vi "USB6343_Control_v1.6.2.vi"(8 "error in":errorcluster caption="错误输出", 10 "interface":T2, 11 "tasks":T3) -> ()   [LabVIEW 2013]
uses:
  <vilib>/DAQmx/read.llb/DAQmx Read (Analog 1D DBL NChan 1Samp).vi
  <vilib>/DAQmx/read.llb/DAQmx Read (Digital 1D Bool NChan 1Samp 1Line).vi
  <vilib>/DAQmx/read.llb/DAQmx Read (Counter DBL 1Chan 1Samp).vi
  <vilib>/DAQmx/write.llb/DAQmx Write (Digital 1D Bool NChan 1Samp 1Line).vi
  <vilib>/DAQmx/write.llb/DAQmx Write (Analog 1D DBL NChan 1Samp).vi
  <vilib>/DAQmx/miscellaneous.llb/DAQmx Fill In Error Info.vi
  <vilib>/DAQmx/configure/timing.llb/DAQmx Timing (Implicit).vi
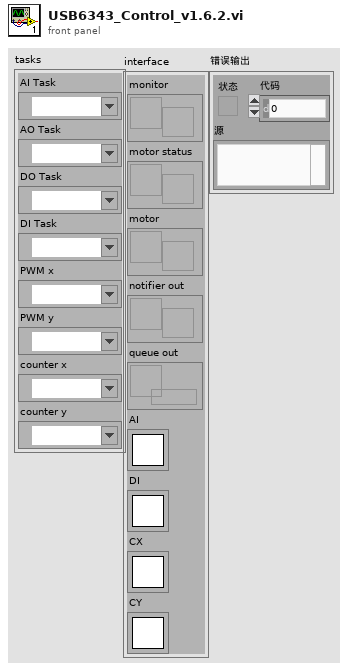
[diagram p1: front panel]
types:
  T1 = typedef "Semaphore RefNum" = refnum<k1>
  T2 = cluster{"monitor":refnum<user-event>, "motor status":refnum<user-event>, "motor":refnum<user-event>, "notifier out":refnum<notifier>, "queue out":refnum<queue>, "AI":T1, "DI":T1, "CX":T1, "CY":T1}
  T3 = cluster{"AI Task":refnum<k21>, "AO Task":refnum<k21>, "DO Task":refnum<k21>, "DI Task":refnum<k21>, "PWM x":refnum<k21>, "PWM y":refnum<k21>, "counter x":refnum<k21>, "counter y":refnum<k21>}
  T4 = cluster{"cmd":string, "channel":i32, "value":dbl, "on/off":bool, "return value":refnum<vi>}
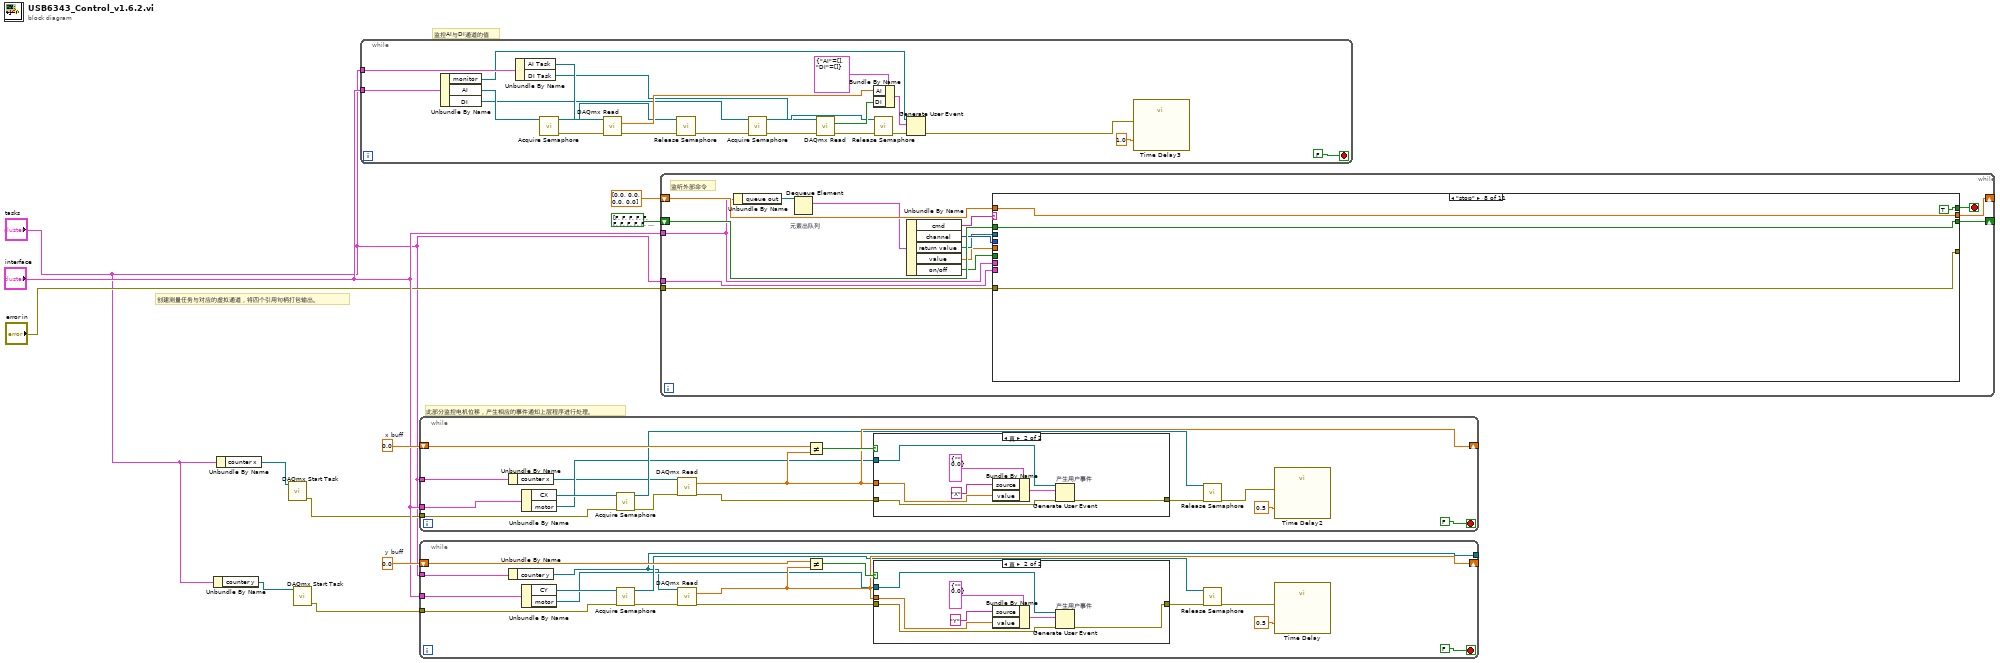
[diagram p0: block diagram]
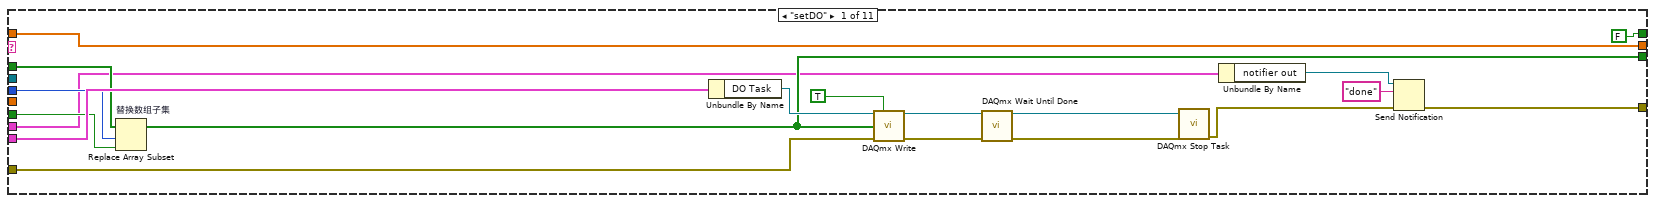
[diagram p4: hidden frame]
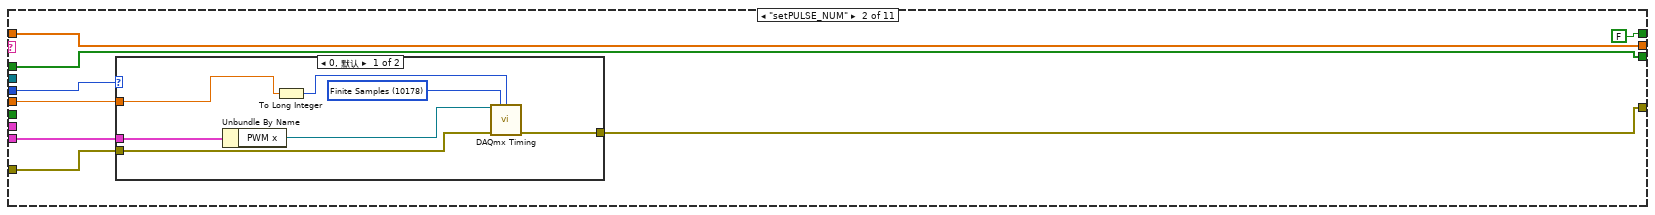
[diagram p5: hidden frame]
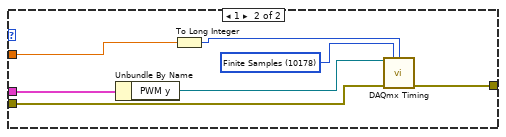
[diagram p6: hidden frame]
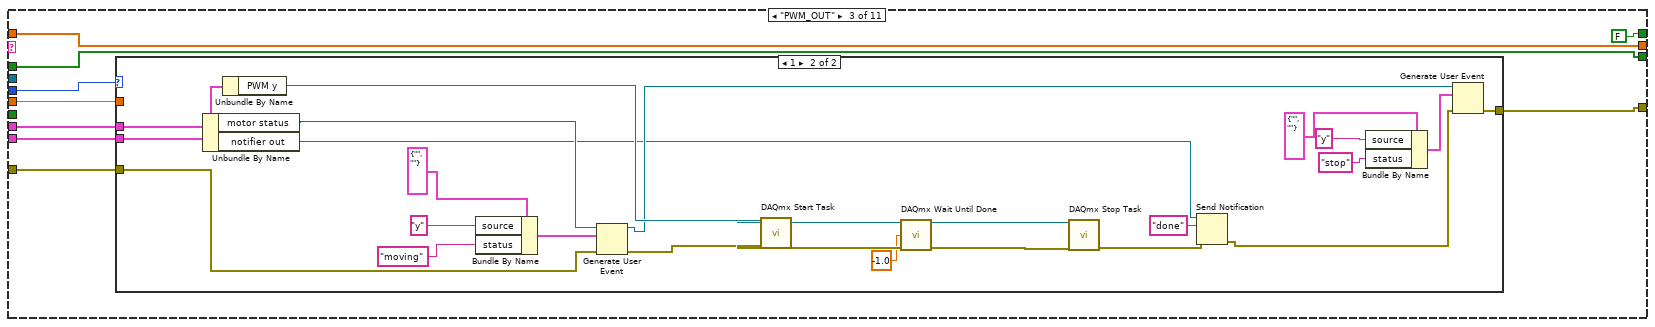
[diagram p7: hidden frame]
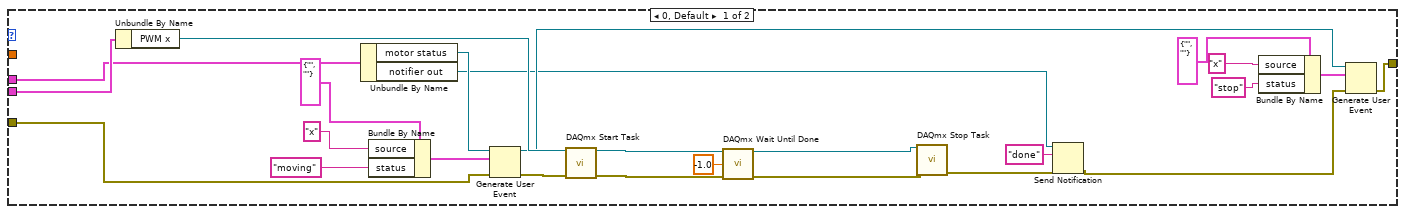
[diagram p8: hidden frame]
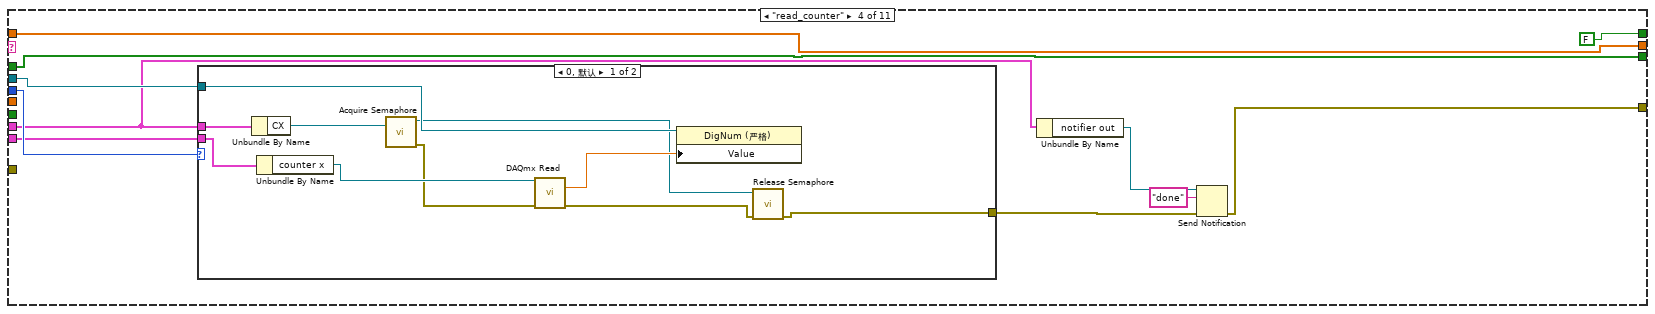
[diagram p9: hidden frame]
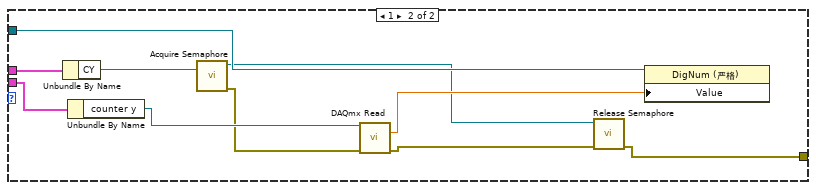
[diagram p10: hidden frame]
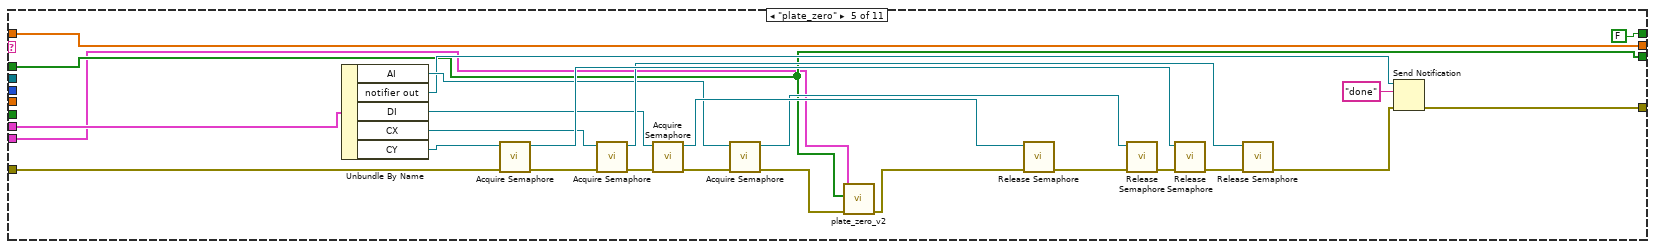
[diagram p11: hidden frame]
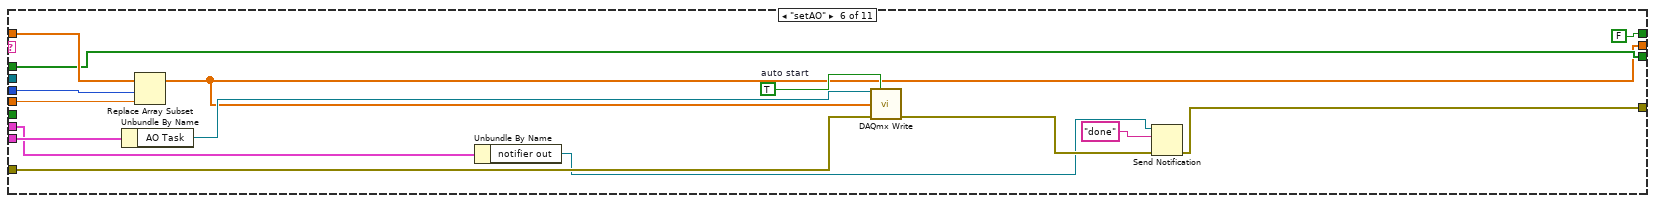
[diagram p12: hidden frame]
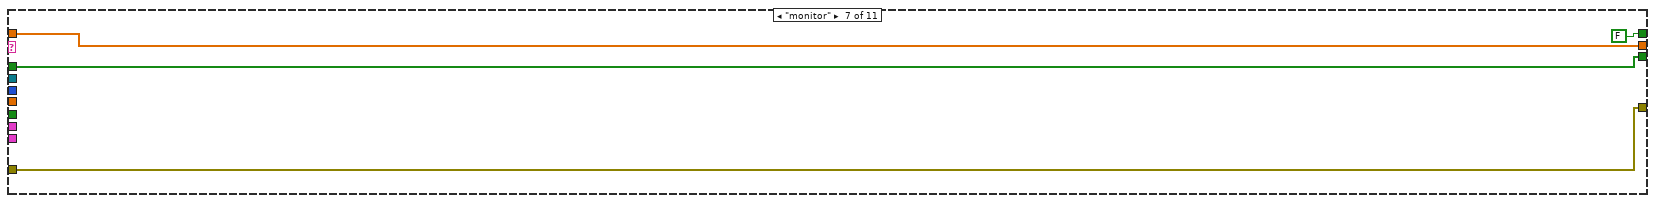
[diagram p13: hidden frame]
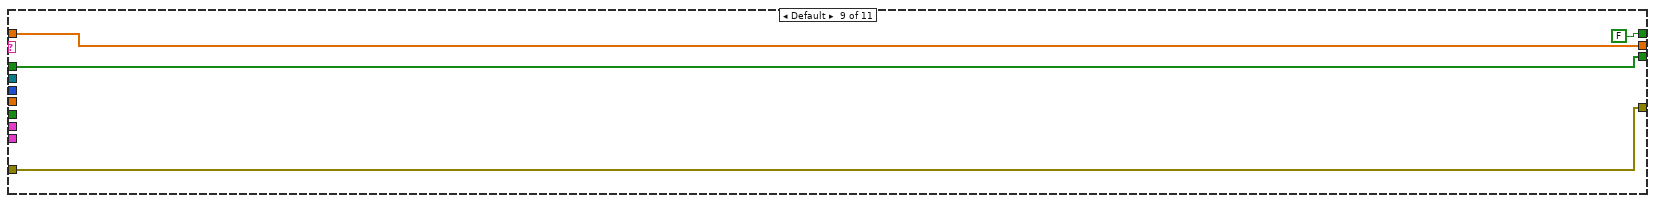
[diagram p14: hidden frame]
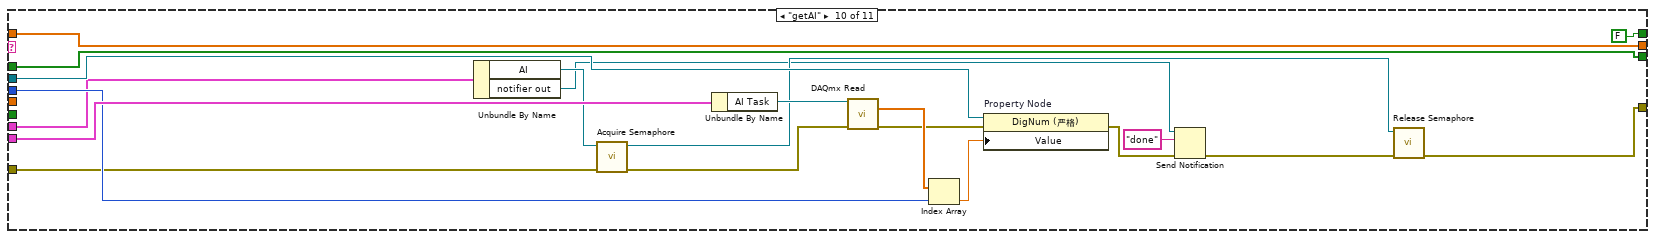
[diagram p15: hidden frame]
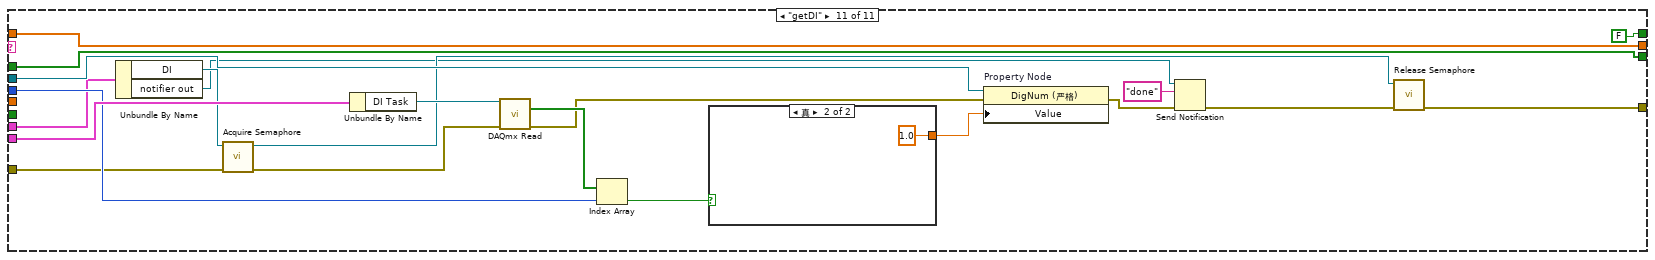
[diagram p16: hidden frame]
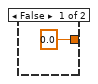
[diagram p17: hidden frame]
diagram:
  w8 = 0.0  # x buff
  w9 = 0.0  # y buff
  # "监控AI与DI通道的值"
  # "此部分监控电机位移，产生相应的事件通知上层程序进行处理。"
  # "创建测量任务与对应的虚拟通道，将四个引用句柄打包输出。"
  n1 = Unbundle By Name("tasks") -> ("counter y"=w1:refnum<k21>)
  n2 = Unbundle By Name("tasks") -> ("counter x"=w3:refnum<k21>)
  n3 = call <vilib>:"DAQmx Start Task.vi"("task/channels in"=w3) -> ("error out"=w4:errorcluster)  [unwired: 13 in, 1 out]
  n4 = call <vilib>:"DAQmx Start Task.vi"("task/channels in"=w1) -> ("error out"=w5:errorcluster)  [unwired: 13 in, 1 out]
  n5 = while {
    tunnel: "tasks" -> [w31]
    tunnel: "interface" -> [w16]
    stop <- FALSE stop-if-true
    n6 = Unbundle By Name(w16) -> ("monitor"=w15:refnum<user-event>, "AI"=w14:T1, "DI"=w13:T1)
    n7 = Unbundle By Name(w31) -> ("AI Task"=w32:refnum<k21>, "DI Task"=w12:refnum<k21>)
    n8 = call <vilib>:"Acquire Semaphore.vi"("semaphore"=w14) -> ("error out"=w17:errorcluster, "semaphore out"=w19:T1)  [unwired: 4 in, 1 out]
    n9 = call-poly <vilib>:"DAQmx Read.vi"("task/channels in"=w32, "error in"=w17) -> ("data"=w29:dbl[], "error out"=w24:errorcluster)  [unwired: 11 in, 1 out]
    n10 = call <vilib>:"Release Semaphore.vi"("error in (no error)"=w24, "semaphore"=w19) -> ("error out"=w23:errorcluster)  [unwired: 4 in, 1 out]
    n11 = call <vilib>:"Acquire Semaphore.vi"("error in (no error)"=w23, "semaphore"=w13) -> ("error out"=w22:errorcluster, "semaphore out"=w18:T1)  [unwired: 3 in, 1 out]
    n12 = call-poly <vilib>:"DAQmx Read.vi"("task/channels in"=w12, "error in"=w22) -> ("data"=w28:bool[], "error out"=w21:errorcluster)  [unwired: 11 in, 1 out]
    n13 = Bundle By Name(cluster=cluster{"AI":dbl[], "DI":bool[]} {"AI"=[], "DI"=[]} ("event data"), "AI"=w29, "DI"=w28) -> (w25:cluster{"AI":dbl[], "DI":bool[]})
    n14 = call <vilib>:"Release Semaphore.vi"("error in (no error)"=w21, "semaphore"=w18) -> ("error out"=w20:errorcluster)  [unwired: 4 in, 1 out]
    n15 = Generate User Event(user event=w15, event data cluster=w25, error in=w20) -> (error out=w27:errorcluster)  [unwired: 1 in, 1 out]
    n16 = call "Time Delay3"("error in (no error)"=w27, "Delay Time (s)"=1.0) -> ()  [unwired: 9 in, 1 out]
  }
  n17 = while {
    shift-right: [w45] -> _
    shift-left: w8 -> [w49]
    tunnel: "interface" -> [w39]
    tunnel: "tasks" -> [w36]
    tunnel: w4 -> [w34]
    stop <- FALSE stop-if-true
    n18 = Unbundle By Name(w36) -> ("counter x"=w35:refnum<k21>)
    n19 = Unbundle By Name(w39) -> ("CX"=w38:T1, "motor"=w37:refnum<user-event>)
    n20 = call <vilib>:"Acquire Semaphore.vi"("error in (no error)"=w34, "semaphore"=w38) -> ("error out"=w44:errorcluster, "semaphore out"=w41:T1)  [unwired: 3 in, 1 out]
    n21 = call-poly <vilib>:"DAQmx Read.vi"("task/channels in"=w35, "error in"=w44) -> ("data"=w45:dbl, "error out"=w47:errorcluster)  [unwired: 11 in, 1 out]
    n22 = Not Equal?(x=w49, y=w45) -> (x != y?=w48:bool)
    n23 = case shown="真" w48 {
      tunnel: w45 -> [_ w51]
      tunnel: w47 -> [w50 w54]
      tunnel: [w50 w53] -> w43
      tunnel: w37 -> [_ w52]
      frame False {
      }
      frame True {
        n24 = Bundle By Name(cluster=cluster{"source":string, "value":dbl} {"source"="", "value"=0.0} ("事件数据"), "source"="X", "value"=w51) -> (w55:cluster{"source":string, "value":dbl})
        n25 = Generate User Event "产生用户事件"(user event=w52, event data cluster=w55, error in=w54) -> (error out=w53:errorcluster)  [unwired: 1 in, 1 out]
      }
    }
    n26 = call <vilib>:"Release Semaphore.vi"("error in (no error)"=w43, "semaphore"=w41) -> ("error out"=w42:errorcluster)  [unwired: 4 in, 1 out]
    n27 = call "Time Delay2"("error in (no error)"=w42, "Delay Time (s)"=0.5) -> ()  [unwired: 9 in, 1 out]
  }
  n28 = while {
    tunnel: [w59] -> _
    shift-right: [w69] -> _
    shift-left: w9 -> [w73]
    tunnel: "interface" -> [w63]
    tunnel: "tasks" -> [w60]
    tunnel: w5 -> [w58]
    stop <- FALSE stop-if-true
    n29 = Unbundle By Name(w60) -> ("counter y"=w59:refnum<k21>)
    n30 = Unbundle By Name(w63) -> ("CY"=w62:T1, "motor"=w61:refnum<user-event>)
    n31 = call <vilib>:"Acquire Semaphore.vi"("error in (no error)"=w58, "semaphore"=w62) -> ("error out"=w68:errorcluster, "semaphore out"=w65:T1)  [unwired: 3 in, 1 out]
    n32 = call-poly <vilib>:"DAQmx Read.vi"("task/channels in"=w59, "error in"=w68) -> ("data"=w69:dbl, "error out"=w71:errorcluster)  [unwired: 11 in, 1 out]
    n33 = Not Equal?(x=w73, y=w69) -> (x != y?=w72:bool)
    n34 = case shown="真" w72 {
      tunnel: w69 -> [_ w75]
      tunnel: w71 -> [w74 w77]
      tunnel: [w74 w76] -> w67
      tunnel: w61 -> [_ w78]
      frame False {
      }
      frame True {
        n35 = Bundle By Name(cluster=cluster{"source":string, "value":dbl} {"source"="", "value"=0.0} ("事件数据"), "source"="Y", "value"=w75) -> (w79:cluster{"source":string, "value":dbl})
        n36 = Generate User Event "产生用户事件"(user event=w78, event data cluster=w79, error in=w77) -> (error out=w76:errorcluster)  [unwired: 1 in, 1 out]
      }
    }
    n37 = call <vilib>:"Release Semaphore.vi"("error in (no error)"=w67, "semaphore"=w65) -> ("error out"=w66:errorcluster)  [unwired: 4 in, 1 out]
    n38 = call "Time Delay"("error in (no error)"=w66, "Delay Time (s)"=0.5) -> ()  [unwired: 9 in, 1 out]
  }
  n39 = while {
    tunnel: "tasks" -> [w90]
    tunnel: "error in" -> [w96]
    shift-right: [w94] -> _
    shift-left: bool[] [FALSE, FALSE, FALSE, FALSE, FALSE, FALSE, FALSE, FALSE, FALSE, FALSE, FALSE, FALSE, FALSE, FALSE, FALSE, FALSE] -> [w95]
    shift-right: [w91] -> _
    shift-left: dbl[] [0.0, 0.0, 0.0, 0.0] ("data") -> [w92]
    tunnel: "interface" -> [w83]
    stop <- w93 stop-if-true
    # "监听外部命令"
    n40 = Unbundle By Name(w83) -> ("queue out"=w82:refnum<queue>)
    n41 = Dequeue Element "元素出队列"(queue=w82) -> (element=w89:T4)  [unwired: 2 in, 3 out]
    n42 = Unbundle By Name(w89) -> ("cmd"=w88:string, "channel"=w87:i32, "return value"=w86:refnum<vi>, "value"=w84:dbl, "on/off"=w85:bool)
    n43 = case shown="\"stop\"" w88 {
      tunnel: w87 -> [w113 w117 w140 w207 _ w266 _ _ _ w296 w319]
      tunnel: w90 -> [w115 w120 w143 w206 w229 w268 _ _ _ w300 w321]
      tunnel: w96 -> [w107 w118 w141 _ w245 w261 w269 w273 w277 w289 w309]
      tunnel: w95 -> [w114 w121 w144 w197 w231 w264 w272 w276 w280 w294 w318]
      tunnel: w85 -> [w112 _ _ _ _ _ _ _ _ _ _]
      tunnel: [w105 w121 w144 w197 w231 w264 w272 w276 w280 w294 w318] -> w94
      tunnel: [FALSE FALSE FALSE FALSE FALSE FALSE FALSE TRUE FALSE FALSE FALSE] -> w93
      tunnel: w92 -> [w110 w122 w145 w198 w252 w265 w271 w274 w278 w293 w317]
      tunnel: [w110 w122 w145 w198 w252 w254 w271 w274 w278 w293 w317] -> w91
      tunnel: w86 -> [_ _ _ w205 _ _ _ _ _ w298 w320]
      tunnel: [w109 w116 w139 w200 w251 w258 w269 w273 w277 w285 w304] -> _
      tunnel: w84 -> [_ w119 w142 _ _ w260 _ _ _ _ _]
      tunnel: w83 -> [w101 _ w138 w203 w237 w257 _ _ _ w283 w303]
      frame "setDO" {
        n44 = Replace Array Subset "替换数组子集"(array=w114, new element=w112, index=w113) -> (w105:bool[])
        n45 = Unbundle By Name(w115) -> ("DO Task"=w106:refnum<k21>)
        n46 = call-poly <vilib>:"DAQmx Write.vi"("task/channels in"=w106, "auto start"=TRUE, "data"=w105, "error in"=w107) -> ("task out"=w102:refnum<k21>, "error out"=w103:errorcluster)  [unwired: 9 in, 1 out]
        n47 = call <vilib>:"DAQmx Wait Until Done.vi"("task/channels in"=w102, "error in"=w103) -> ("task out"=w97:refnum<k21>, "error out"=w99:errorcluster)  [unwired: 12 in]
        n48 = call <vilib>:"DAQmx Stop Task.vi"("task/channels in"=w97, "error in"=w99) -> ("error out"=w98:errorcluster)  [unwired: 12 in, 1 out]
        n49 = Unbundle By Name(w101) -> ("notifier out"=w100:refnum<notifier>)
        n50 = Send Notification(notification="done" ("通知"), notifier=w100, error in (no error)=w98) -> (error out=w109:errorcluster)  [unwired: 1 out]
      }
      frame "setPULSE_NUM" {
        n51 = case shown="0, 默认" w117 {
          tunnel: w120 -> [w130 w137]
          tunnel: w119 -> [w125 w132]
          tunnel: w118 -> [w127 w134]
          tunnel: [w126 w133] -> w116
          frame 0, Default {
            w128 = 10178 items=["Finite Samples"=10178, "Continuous Samples"=10123, "Hardware Timed Single Point"=12522] ("sample mode")
            n52 = Unbundle By Name(w130) -> ("PWM x"=w129:refnum<k21>)
            n53 = To Long Integer(number=w125) -> (32bit integer=w124:i32)
            n54 = call-poly <vilib>:"DAQmx Timing.vi"("task/channels in"=w129, "sample mode"=w128, "samples per channel"=w124, "error in"=w127) -> ("error out"=w126:errorcluster)  [unwired: 10 in, 1 out]
          }
          frame 1 {
            w135 = 10178 items=["Finite Samples"=10178, "Continuous Samples"=10123, "Hardware Timed Single Point"=12522] ("sample mode")
            n55 = Unbundle By Name(w137) -> ("PWM y"=w136:refnum<k21>)
            n56 = To Long Integer(number=w132) -> (32bit integer=w131:i32)
            n57 = call-poly <vilib>:"DAQmx Timing.vi"("task/channels in"=w136, "sample mode"=w135, "samples per channel"=w131, "error in"=w134) -> ("error out"=w133:errorcluster)  [unwired: 10 in, 1 out]
          }
        }
      }
      frame "PWM_OUT" {
        n58 = case shown="1" w140 {
          tunnel: w143 -> [w171 w196]
          tunnel: w142 -> [_ _]
          tunnel: w141 -> [w163 w188]
          tunnel: [w156 w182] -> w139
          tunnel: w138 -> [w154 w179]
          frame 0, Default {
            n59 = Unbundle By Name(w171) -> ("PWM x"=w170:refnum<k21>)
            n60 = Unbundle By Name(w154) -> ("motor status"=w153:refnum<user-event>, "notifier out"=w148:refnum<notifier>)
            n61 = Bundle By Name(cluster=cluster{"source":string, " status":string} {"source"="", " status"=""} ("event data"), "source"="x", "status"="moving") -> (w161:cluster{"source":string, " status":string})
            n62 = Generate User Event(user event=w153, event data cluster=w161, error in=w163) -> (user event out=w155:refnum<user-event>, error out=w162:errorcluster)  [unwired: 1 in]
            n63 = call <vilib>:"DAQmx Start Task.vi"("task/channels in"=w170, "error in"=w162) -> ("task out"=w168:refnum<k21>, "error out"=w169:errorcluster)  [unwired: 12 in]
            n64 = call <vilib>:"DAQmx Wait Until Done.vi"("task/channels in"=w168, "timeout (sec)"=-1.0, "error in"=w169) -> ("task out"=w167:refnum<k21>, "error out"=w152:errorcluster)  [unwired: 11 in]
            n65 = call <vilib>:"DAQmx Stop Task.vi"("task/channels in"=w167, "error in"=w152) -> ("error out"=w151:errorcluster)  [unwired: 12 in, 1 out]
            n66 = Send Notification(notification="done", notifier=w148, error in (no error)=w151) -> (error out=w150:errorcluster)  [unwired: 1 out]
            n67 = Bundle By Name(cluster=cluster{"source":string, " status":string} {"source"="", " status"=""} ("event data"), "source"="x", "status"="stop") -> (w157:cluster{"source":string, " status":string})
            n68 = Generate User Event(user event=w155, event data cluster=w157, error in=w150) -> (error out=w156:errorcluster)  [unwired: 1 in, 1 out]
          }
          frame 1 {
            n69 = Unbundle By Name(w179) -> ("motor status"=w178:refnum<user-event>, "notifier out"=w173:refnum<notifier>)
            n70 = Unbundle By Name(w196) -> ("PWM y"=w195:refnum<k21>)
            n71 = Bundle By Name(cluster=cluster{"source":string, " status":string} {"source"="", " status"=""} ("event data"), "source"="y", "status"="moving") -> (w181:cluster{"source":string, " status":string})
            n72 = Generate User Event(user event=w178, event data cluster=w181, error in=w188) -> (user event out=w177:refnum<user-event>, error out=w187:errorcluster)  [unwired: 1 in]
            n73 = call <vilib>:"DAQmx Start Task.vi"("task/channels in"=w195, "error in"=w187) -> ("task out"=w193:refnum<k21>, "error out"=w194:errorcluster)  [unwired: 12 in]
            n74 = call <vilib>:"DAQmx Wait Until Done.vi"("task/channels in"=w193, "timeout (sec)"=-1.0, "error in"=w194) -> ("task out"=w191:refnum<k21>, "error out"=w192:errorcluster)  [unwired: 11 in]
            n75 = call <vilib>:"DAQmx Stop Task.vi"("task/channels in"=w191, "error in"=w192) -> ("error out"=w176:errorcluster)  [unwired: 12 in, 1 out]
            n76 = Send Notification(notification="done", notifier=w173, error in (no error)=w176) -> (error out=w175:errorcluster)  [unwired: 1 out]
            n77 = Bundle By Name(cluster=cluster{"source":string, " status":string} {"source"="", " status"=""} ("event data"), "source"="y", "status"="stop") -> (w183:cluster{"source":string, " status":string})
            n78 = Generate User Event(user event=w177, event data cluster=w183, error in=w175) -> (error out=w182:errorcluster)  [unwired: 1 in, 1 out]
          }
        }
      }
      frame "read_counter" {
        n79 = case shown="0, 默认" w207 {
          tunnel: w203 -> [w217 w227]
          tunnel: w206 -> [w215 w225]
          tunnel: w205 -> [w212 w222]
          tunnel: [w208 w218] -> w204
          frame 0, Default {
            n80 = Unbundle By Name(w217) -> ("CX"=w216:T1)
            n81 = Unbundle By Name(w215) -> ("counter x"=w214:refnum<k21>)
            n82 = call <vilib>:"Acquire Semaphore.vi"("semaphore"=w216) -> ("error out"=w213:errorcluster, "semaphore out"=w209:T1)  [unwired: 4 in, 1 out]
            n83 = call-poly <vilib>:"DAQmx Read.vi"("task/channels in"=w214, "error in"=w213) -> ("data"=w211:dbl, "error out"=w210:errorcluster)  [unwired: 11 in, 1 out]
            n84 = property class="DigNum (严格)"(reference=w212, "Value"=w211) -> ()  [unwired: 1 in, 2 out]
            n85 = call <vilib>:"Release Semaphore.vi"("error in (no error)"=w210, "semaphore"=w209) -> ("error out"=w208:errorcluster)  [unwired: 4 in, 1 out]
          }
          frame 1 {
            n86 = Unbundle By Name(w227) -> ("CY"=w226:T1)
            n87 = Unbundle By Name(w225) -> ("counter y"=w224:refnum<k21>)
            n88 = call <vilib>:"Acquire Semaphore.vi"("semaphore"=w226) -> ("error out"=w223:errorcluster, "semaphore out"=w219:T1)  [unwired: 4 in, 1 out]
            n89 = call-poly <vilib>:"DAQmx Read.vi"("task/channels in"=w224, "error in"=w223) -> ("data"=w221:dbl, "error out"=w220:errorcluster)  [unwired: 11 in, 1 out]
            n90 = call <vilib>:"Release Semaphore.vi"("error in (no error)"=w220, "semaphore"=w219) -> ("error out"=w218:errorcluster)  [unwired: 4 in, 1 out]
            n91 = property class="DigNum (严格)"(reference=w222, "Value"=w221) -> ()  [unwired: 1 in, 2 out]
          }
        }
        n92 = Unbundle By Name(w203) -> ("notifier out"=w202:refnum<notifier>)
        n93 = Send Notification(notification="done", notifier=w202, error in (no error)=w204) -> (error out=w200:errorcluster)  [unwired: 1 out]
      }
      frame "plate_zero" {
        n94 = Unbundle By Name(w237) -> ("AI"=w236:T1, "notifier out"=w232:refnum<notifier>, "DI"=w235:T1, "CX"=w234:T1, "CY"=w233:T1)
        n95 = call <vilib>:"Acquire Semaphore.vi"("error in (no error)"=w245, "semaphore"=w233) -> ("error out"=w247:errorcluster, "semaphore out"=w241:T1)  [unwired: 3 in, 1 out]
        n96 = call <vilib>:"Acquire Semaphore.vi"("error in (no error)"=w247, "semaphore"=w234) -> ("error out"=w246:errorcluster, "semaphore out"=w238:T1)  [unwired: 3 in, 1 out]
        n97 = call <vilib>:"Acquire Semaphore.vi"("error in (no error)"=w246, "semaphore"=w235) -> ("error out"=w249:errorcluster, "semaphore out"=w240:T1)  [unwired: 3 in, 1 out]
        n98 = call <vilib>:"Acquire Semaphore.vi"("error in (no error)"=w249, "semaphore"=w236) -> ("error out"=w230:errorcluster, "semaphore out"=w239:T1)  [unwired: 3 in, 1 out]
        n99 = call "plate_zero_v2.vi"("error in"=w230, "DO array"=w231, "tasks"=w229) -> ("error out"=w228:errorcluster)  [unwired: 8 in]
        n100 = call <vilib>:"Release Semaphore.vi"("error in (no error)"=w228, "semaphore"=w240) -> ("error out"=w248:errorcluster)  [unwired: 4 in, 1 out]
        n101 = call <vilib>:"Release Semaphore.vi"("error in (no error)"=w248, "semaphore"=w239) -> ("error out"=w244:errorcluster)  [unwired: 4 in, 1 out]
        n102 = call <vilib>:"Release Semaphore.vi"("error in (no error)"=w244, "semaphore"=w241) -> ("error out"=w243:errorcluster)  [unwired: 4 in, 1 out]
        n103 = call <vilib>:"Release Semaphore.vi"("error in (no error)"=w243, "semaphore"=w238) -> ("error out"=w242:errorcluster)  [unwired: 4 in, 1 out]
        n104 = Send Notification(notification="done", notifier=w232, error in (no error)=w242) -> (error out=w251:errorcluster)  [unwired: 1 out]
      }
      frame "setAO" {
        w263 = TRUE  # auto start
        n105 = Unbundle By Name(w268) -> ("AO Task"=w267:refnum<k21>)
        n106 = Replace Array Subset(array=w265, new element=w260, index=w266) -> (w254:dbl[])
        n107 = Unbundle By Name(w257) -> ("notifier out"=w256:refnum<notifier>)
        n108 = call-poly <vilib>:"DAQmx Write.vi"("task/channels in"=w267, "auto start"=w263, "data"=w254, "error in"=w261) -> ("error out"=w259:errorcluster)  [unwired: 9 in, 2 out]
        n109 = Send Notification(notification="done", notifier=w256, error in (no error)=w259) -> (error out=w258:errorcluster)  [unwired: 1 out]
      }
      frame "monitor" {
      }
      frame "stop" {
      }
      frame Default {
      }
      frame "getAI" {
        n110 = Unbundle By Name(w283) -> ("AI"=w282:T1, "notifier out"=w281:refnum<notifier>)
        n111 = call <vilib>:"Acquire Semaphore.vi"("error in (no error)"=w289, "semaphore"=w282) -> ("error out"=w288:errorcluster, "semaphore out"=w284:T1)  [unwired: 3 in, 1 out]
        n112 = Unbundle By Name(w300) -> ("AI Task"=w299:refnum<k21>)
        n113 = call-poly <vilib>:"DAQmx Read.vi"("task/channels in"=w299, "error in"=w288) -> ("data"=w297:dbl[], "error out"=w287:errorcluster)  [unwired: 11 in, 1 out]
        n114 = Index Array(array=w297, index=w296) -> (element=w295:dbl)
        n115 = property on="Property Node" class="DigNum (严格)"(reference=w298, error in=w287, "Value"=w295) -> (error out=w290:errorcluster)  [unwired: 1 out]
        n116 = Send Notification(notification="done" ("通知"), notifier=w281, error in (no error)=w290) -> (error out=w286:errorcluster)  [unwired: 1 out]
        n117 = call <vilib>:"Release Semaphore.vi"("error in (no error)"=w286, "semaphore"=w284) -> ("error out"=w285:errorcluster)  [unwired: 4 in, 1 out]
      }
      frame "getDI" {
        n118 = Unbundle By Name(w303) -> ("DI"=w302:T1, "notifier out"=w301:refnum<notifier>)
        n119 = call <vilib>:"Acquire Semaphore.vi"("error in (no error)"=w309, "semaphore"=w302) -> ("error out"=w308:errorcluster, "semaphore out"=w305:T1)  [unwired: 3 in, 1 out]
        n120 = Unbundle By Name(w321) -> ("DI Task"=w313:refnum<k21>)
        n121 = call-poly <vilib>:"DAQmx Read.vi"("task/channels in"=w313, "error in"=w308) -> ("data"=w312:bool[], "error out"=w307:errorcluster)  [unwired: 11 in, 1 out]
        n122 = Index Array "Index Array"(array=w312, index=w319) -> (element=w311:bool)
        n123 = case shown="真" w311 {
          tunnel: [0.0 1.0] -> w310
          frame False {
          }
          frame True {
          }
        }
        n124 = property on="Property Node" class="DigNum (严格)"(reference=w320, error in=w307, "Value"=w310) -> (error out=w314:errorcluster)  [unwired: 1 out]
        n125 = Send Notification(notification="done" ("通知"), notifier=w301, error in (no error)=w314) -> (error out=w306:errorcluster)  [unwired: 1 out]
        n126 = call <vilib>:"Release Semaphore.vi"("error in (no error)"=w306, "semaphore"=w305) -> ("error out"=w304:errorcluster)  [unwired: 4 in, 1 out]
      }
    }
  }
